vi "Write Tx.vi"(8 "error in (no error)":errorcluster, 10 "Tx":refnum<queue>, 11 "RxTx in":refnum<class "CM_RxTx.lvclass">) -> (0 "error out":errorcluster, 3 "RxTx out":refnum<class "CM_RxTx.lvclass">)   [LabVIEW 2018, in "CM_RxTx.lvclass"]
uses:
  CM_RxTx.lvclass
  CM_RxTx.lvclass/CM_RxTx.ctl
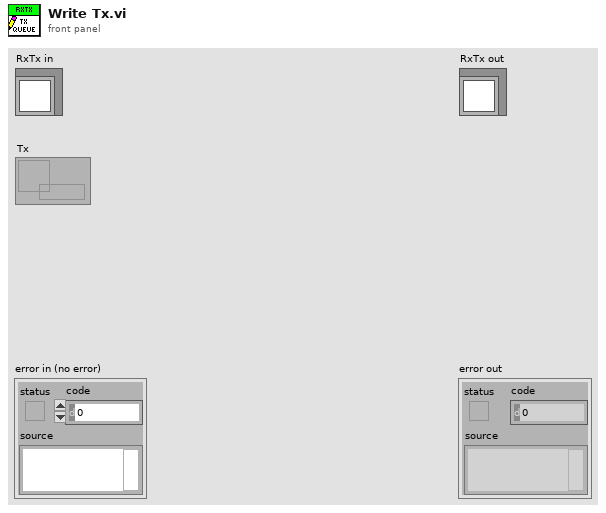
[diagram p1: front panel]
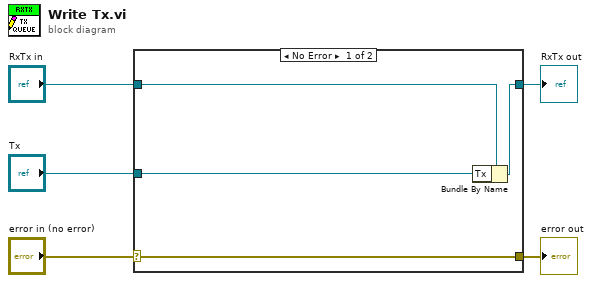
[diagram p0: block diagram]
diagram:
  n1 = case shown="No Error" "error in (no error)" {
    selector: "error in (no error)" -> [w9 w10]
    tunnel: [w9 w10] -> w4
    tunnel: [w7 w11] -> w2
    tunnel: "RxTx in" -> [w8 w11]
    tunnel: "Tx" -> [w6 _]
    frame No Error {
      n2 = Bundle By Name(cluster=w8, "Tx"=w6) -> (w7:refnum<class "CM_RxTx.lvclass">)
    }
    frame Error {
    }
  }
  "error out" <- w4
  "RxTx out" <- w2
